vi "example_moveTerminal.vi"() -> ()   [LabVIEW 2023]
uses:
  Ctrls/direction.ctl
  Terminal/Terminal.lvclass
  BlockDiagram/Read controlTerminals.vi
  GObject/Read bounds.vi
  TLC_Scripto.lvlib
  BlockDiagram/BlockDiagram.lvclass
panel:
  in  "horizontalShift":i32(slide) scale=-60.0..140.0
  in  "verticalShift":i32(slide) scale=-84.0..116.0
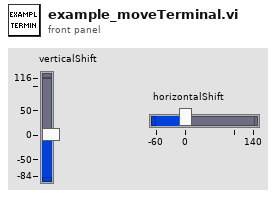
[diagram p1: front panel]
types:
  T1 = typedef "LVBoundsTypeDef.ctl" = cluster{"Width":u32, "Height":u32}
  T2 = typedef "TLC_Scripto.lvlib/direction.ctl" = enum16{"Horizontal", "Vertical"}
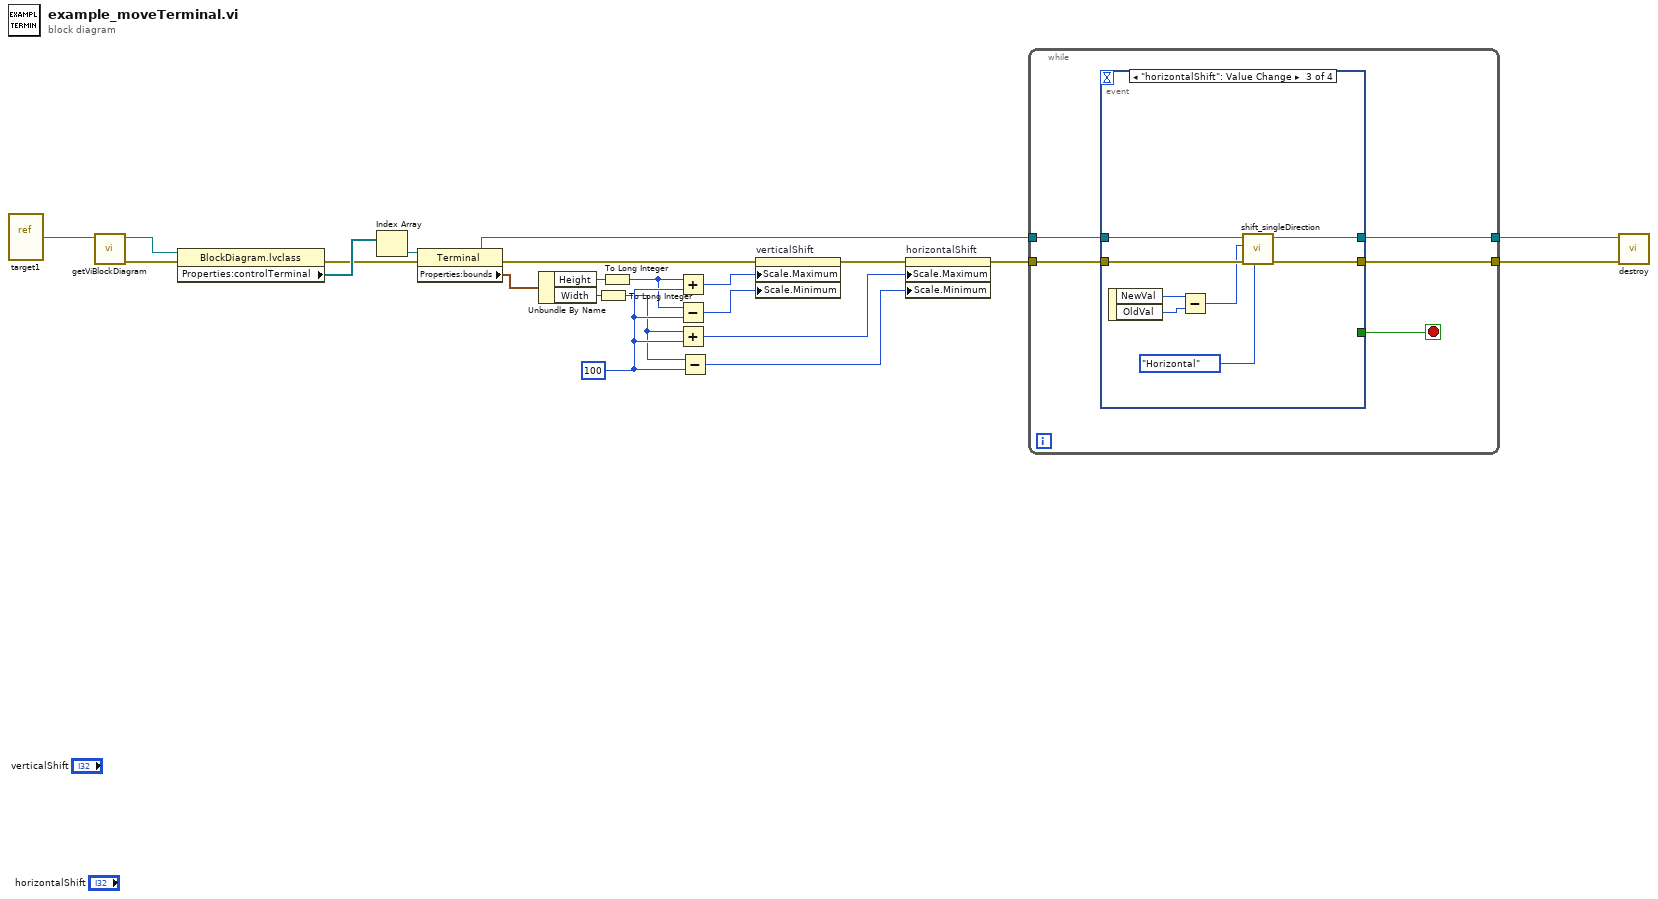
[diagram p0: block diagram]
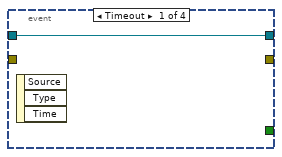
[diagram p2: hidden frame]
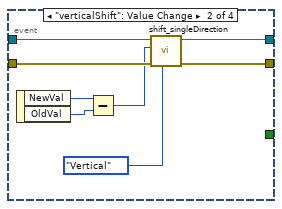
[diagram p3: hidden frame]
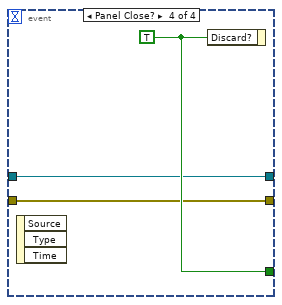
[diagram p4: hidden frame]
diagram:
  w10 = 100 ("y")
  n1 = vi-ref "target1.vi"() -> (w22:refnum<vi>)
  n2 = call "getViBlockDiagram.vi"("ViRef"=w22) -> ("error out"=w21:errorcluster, "topMostBlockDiagram"=w20:refnum<class "BlockDiagram.lvclass">)  [unwired: 9 in]
  n3 = property class="BlockDiagram.lvclass"(reference=w20, error in=w21) -> (error out=w7:errorcluster, "Properties:controlTerminal"=w19:refnum<class "Terminal.lvclass">[])  [unwired: 1 out]
  n4 = Index Array(array=w19) -> (element=w18:refnum<class "Terminal.lvclass">)  [unwired: 1 in]
  n5 = property class="Terminal"(reference=w18, error in=w7) -> (reference out=w5:refnum<class "Terminal.lvclass">, error out=w6:errorcluster, "Properties:bounds"=w17:T1)
  n6 = Unbundle By Name(w17) -> ("Height"=w16:u32, "Width"=w11:u32)
  n7 = To Long Integer(number=w11) -> (32bit integer=w1:i32)
  n8 = To Long Integer(number=w16) -> (32bit integer=w2:i32)
  n9 = Add(x=w2, y=w10) -> (x+y=w15:i32)
  n10 = Subtract(x=w2, y=w10) -> (x-y=w14:i32)
  n11 = Add(x=w1, y=w10) -> (x+y=w12:i32)
  n12 = Subtract(x=w1, y=w10) -> (x-y=w9:i32)
  n13 = property on="verticalShift" class="Slide (strict)"(error in=w6, "Scale.Maximum"=w15, "Scale.Minimum"=w14) -> (error out=w13:errorcluster)  [unwired: 1 in, 1 out]
  n14 = property on="horizontalShift" class="Slide (strict)"(error in=w13, "Scale.Maximum"=w12, "Scale.Minimum"=w9) -> (error out=w8:errorcluster)  [unwired: 1 in, 1 out]
  n15 = while {
    tunnel: w8 -> [w26]
    tunnel: w5 -> [w24]
    tunnel: [w23] -> w4
    tunnel: [w25] -> w3
    stop <- w27 stop-if-true
    n16 = event shown="[2] \"horizontalShift\": Value Change" {
      selector: _ -> [_ _ _ _]
      dyn-events: _ -> [_ _ _ _]
      timeout: _ -> [_ _ _ _]
      tunnel: [_ _ _ w47] -> w27
      tunnel: w26 -> [_ w34 w42 w46]
      tunnel: [_ w33 w41 w46] -> w25
      tunnel: w24 -> [w28 w35 w43 w45]
      tunnel: [w28 w36 w44 w45] -> w23
      event Timeout {
        n17 = event-data() -> ()  [unwired: 1 in, 3 out]
      }
      event "verticalShift": Value Change {
        n18 = event-data() -> ("NewVal"=w31:i32, "OldVal"=w30:i32)  [unwired: 1 in]
        n19 = Subtract(x=w31, y=w30) -> (x-y=w29:i32)
        n20 = call-dynamic "shift_singleDirection.vi"("direction"=direction."Vertical", "error in (no error)"=w34, "delta[pixel]"=w29, "GObject in"=w35) -> ("error out"=w33:errorcluster, "GObject out"=w36:refnum<class "Terminal.lvclass">)  [unwired: 6 in]
      }
      event "horizontalShift": Value Change {
        n21 = event-data() -> ("NewVal"=w39:i32, "OldVal"=w38:i32)  [unwired: 1 in]
        n22 = Subtract(x=w39, y=w38) -> (x-y=w37:i32)
        n23 = call-dynamic "shift_singleDirection.vi"("direction"=direction."Horizontal", "error in (no error)"=w42, "delta[pixel]"=w37, "GObject in"=w43) -> ("error out"=w41:errorcluster, "GObject out"=w44:refnum<class "Terminal.lvclass">)  [unwired: 6 in]
      }
      event Panel Close? {
        w47 = TRUE ("Discard?")
        n24 = event-data() -> ()  [unwired: 1 in, 3 out]
        n25 = event-data("Discard?"=w47) -> ()  [unwired: 1 in, 1 out]
      }
    }
  }
  n26 = call-dynamic "destroy.vi"("Error In"=w3, "Generic In"=w4) -> ()  [unwired: 9 in, 1 out]
